vi "IMAQController.AddToLoggerString.vi"(0 "Error Logger In":string, 1 "Buffer size":i32, 2 "Message":string, 3 "Selector":string, 5 "error in":errorcluster) -> (14 "Error Logger Out":string, 16 "Number of lines":i16, 17 "Length of lines":i32[](array[numeric]), 18 "new lines at":i32[](array[numeric]), 19 "error out":errorcluster)   [LabVIEW 2014, in "IMAQController.lvlib"]
uses:
  IMAQController.lvlib
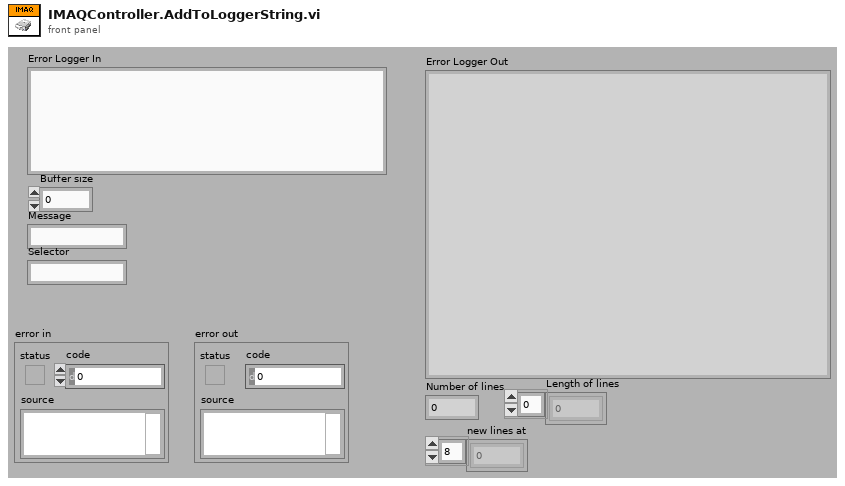
[diagram p1: front panel]
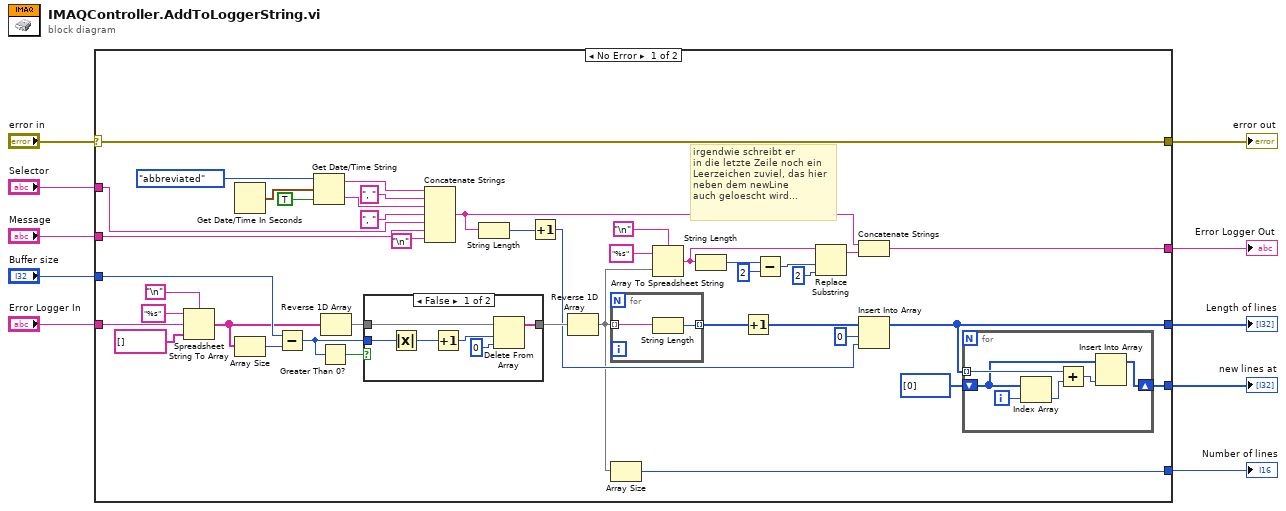
[diagram p0: block diagram]
diagram:
  n1 = case shown="No Error" "error in" {
    selector: "error in" -> [w34 w68]
    tunnel: "Selector" -> [w40 _]
    tunnel: "Message" -> [w39 _]
    tunnel: "Buffer size" -> [w50 _]
    tunnel: [w34 w68] -> w6
    tunnel: "Error Logger In" -> [w36 _]
    tunnel: [w33 _] -> w2
    tunnel: [w11 _] -> w4
    tunnel: [w20 _] -> w1
    tunnel: [w18 _] -> w3
    frame No Error {
      # "irgendwie schreibt er\nin die letzte Zeile noch ein \nLeerzeichen zuviel, das hier\nneben dem newLine\nauch geloescht wird..."
      n2 = Spreadsheet String To Array(delimiter (Tab)="\n", format string="%s", spreadsheet string=w36, array type (2D Dbl)=string[] []) -> (array=w27:string[])
      n3 = Get Date/Time In Seconds() -> (seconds since 1Jan1904=w47:timestamp)
      n4 = Array Size(array=w27) -> (size(s)=w35:i32)
      n5 = Subtract(x=w50, y=w35) -> (x-y=w48:i32)
      n6 = Get Date/Time String(date format (0)=enum16{"short", "long", "abbreviated"}."abbreviated", seconds (now)=w47, want seconds? (F)=TRUE) -> (date string=w44:string, time string=w43:string)
      n7 = Greater Than 0?(x=w48) -> (x > 0?=w49:bool)
      n8 = Reverse 1D Array(array=w27) -> (reversed array=w26:string[])
      n9 = case shown="False" w49 {
        tunnel: w26 -> [w66 w67]
        tunnel: w48 -> [w65 _]
        tunnel: [w62 w67] -> w32
        frame False {
          n10 = Absolute Value(x=w65) -> (abs(x)=w64:i32)
          n11 = Increment(x=w64) -> (x+1=w63:i32)
          n12 = Delete From Array(array=w66, length=w63, index=0) -> (array with subset deleted=w62:string[])  [unwired: 1 out]
        }
        frame True {
        }
      }
      n13 = Concatenate Strings(w44, ", " ("string"), w43, ", " ("string"), w40, w39, "\n") -> (w24:string)
      n14 = String Length(string=w24) -> (length=w23:i32)
      n15 = Increment(x=w23) -> (x+1=w21:i32)
      n16 = Reverse 1D Array(array=w32) -> (reversed array=w17:string[])
      n17 = for {
        tunnel: w17 -> [w60] mode=indexing
        tunnel: [w59] -> w25 mode=indexing
        n18 = String Length(string=w60) -> (length=w59:i32)
      }
      n19 = Array Size(array=w17) -> (size(s)=w11:i32)
      n20 = Array To Spreadsheet String(delimiter (Tab)="\n", array=w17, 3:"%s" ("format string")) -> (spreadsheet string=w16:string)
      n21 = String Length(string=w16) -> (length=w15:i32)
      n22 = Increment(x=w25) -> (x+1=w22:i32[])
      n23 = Subtract(x=w15, y=2) -> (x-y=w14:i32)
      n24 = Replace Substring(2:2 ("length (len. of substring)"), 3:w14, 5:w16) -> (1:w28:string)  [unwired: 1 in, 1 out]
      n25 = Concatenate Strings(w24, w28) -> (w33:string)
      n26 = Insert Into Array(array=w22, index=0, new element=w21) -> (w20:i32[])
      n27 = for {
        tunnel: w20 -> [w58] mode=indexing
        shift-right: [w54] -> w18
        shift-left: i32[] [0] -> [w55]
        i -> [w57]
        n28 = Index Array(array=w55, index=w57) -> (element=w56:i32)
        n29 = Add(x=w58, y=w56) -> (x+y=w53:i32)
        n30 = Insert Into Array(array=w55, new element=w53) -> (w54:i32[])  [unwired: 1 in]
      }
    }
    frame Error {
    }
  }
  "error out" <- w6
  "Error Logger Out" <- w2
  "Number of lines" <- w4
  "Length of lines" <- w1
  "new lines at" <- w3
